vi "Value Change.vi"   [LabVIEW 2020, in "_Template.lvlib" / "Templates.lvlib" / "TEMPLATE jettl Actor.lvlib" / "TEMPLATE Actor.lvlib" / "TEMPLATE Refs.lvlib"]
uses:
  TEMPLATE Refs.lvlib
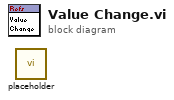
[diagram p0: block diagram]
diagram:
  n1 = call "placeholder.vi"() -> ()  [unwired: 12 in]
